vi "Get World Map.vi"(11 "AnytimeDStar in":refnum<class "NI_Robotics_AnytimeDStar.lvclass">) -> (2 "world map ref in":refnum<data-value>, 3 "AnytimeDStar out":refnum<class "NI_Robotics_AnytimeDStar.lvclass">)   [LabVIEW 2017, in "NI_Robotics_AnytimeDStar.lvclass"]
uses:
  <vilib>/robotics/Navigation/Anytime D Star/NI_Robotics_AnytimeDStar.lvclass
  <vilib>/robotics/Navigation/shared/WorldMap/AbstractDstarWorldMap/NI_Robotics_AbstractDstarWorldMap.lvclass
  <vilib>/robotics/Navigation/Anytime D Star/NI_Robotics_AnytimeDStar.lvclass/NI_Robotics_AnytimeDStar.ctl
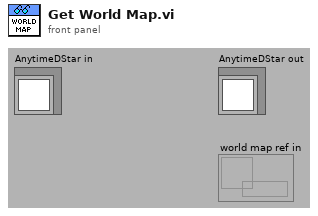
[diagram p1: front panel]
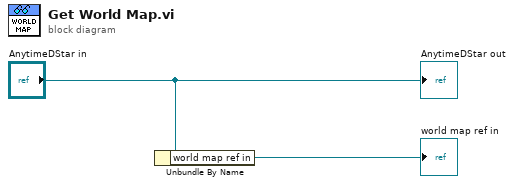
[diagram p0: block diagram]
diagram:
  n1 = Unbundle By Name("AnytimeDStar in") -> ("world map ref in"=→"world map ref in":refnum<data-value>)
  "AnytimeDStar out" <- "AnytimeDStar in"
